vi "AssemblerLauncher.vi"() -> (0 "error out":errorcluster)   [LabVIEW 2017]
uses:
  <vilib>/ActorFramework/Message Enqueuer/Message Priority.ctl
  <vilib>/gpm_packages/@cs/mva-viewable/Source/IViewable/IViewable/View Position Enum.ctl
  <vilib>/gpm_packages/@cs/example/Dynamic Viewables/SequenceSteps/SineModel/SineModel.lvclass
  C:/Program Files/National Instruments/LabVIEW 2017/vi.lib/gpm_packages/@cs/mva-core/Source/IModel/IModel/IModel.lvclass
  <vilib>/gpm_packages/@cs/mva-core/Source/MonitoredMediator/MonitoredMediator/MonitoredMediator.lvclass
  C:/Program Files/National Instruments/LabVIEW 2017/vi.lib/gpm_packages/@cs/mva-core/Source/Mediator/Mediator/Mediator.lvclass
  C:/Program Files/National Instruments/LabVIEW 2017/vi.lib/gpm_packages/@cs/mva-core/Source/IMediator/IMediator/IMediator.lvclass
  <vilib>/gpm_packages/@cs/example/Dynamic Viewables/ViewableChart/ViewableChart.lvclass
  C:/Program Files/National Instruments/LabVIEW 2017/vi.lib/gpm_packages/@cs/mva-viewable/Source/IViewable/IViewable/IViewable.lvclass
  <vilib>/gpm_packages/@cs/example/Dynamic Viewables/ViewableLEDs/ViewableLEDs.lvclass
  <vilib>/gpm_packages/@cs/example/Dynamic Viewables/ViewableButtons/ViewableButtons.lvclass
  <vilib>/gpm_packages/@cs/example/Dynamic Viewables/ViewableStatusBar/ViewableStatusBar.lvclass
  <vilib>/gpm_packages/@cs/example/Dynamic Viewables/SequencingModel/SequencingModel.lvclass
  C:/Program Files/National Instruments/LabVIEW 2017/vi.lib/gpm_packages/@cs/mva-core/Source/IObserver/IObserver/IObserver.lvclass
  <vilib>/gpm_packages/@cs/example/Dynamic Viewables/SequenceSteps/RandomNumberModel/RandomNumberModel.lvclass
  <vilib>/gpm_packages/@cs/example/Dynamic Viewables/SequenceSteps/BlinkyLightModel/BlinkyLightModel.lvclass
  <vilib>/gpm_packages/@cs/example/Dynamic Viewables/ExampleViewModel/ExampleViewModel.lvclass
  C:/Program Files/National Instruments/LabVIEW 2017/vi.lib/gpm_packages/@cs/mva-viewable/Source/IViewModel/IViewModel/IViewModel.lvclass
  C:/Program Files/National Instruments/LabVIEW 2017/vi.lib/ActorFramework/Actor/Actor.lvclass
  <vilib>/gpm_packages/@cs/BusMonitor/ListboxBusMonitor/ListboxBusMonitor/ListboxBusMonitor.lvclass/ListboxBusMonitor.ctl
  <vilib>/gpm_packages/@cs/example/Dynamic Viewables/SequencingModel/SequencingModel.lvclass/SequencingModel.ctl
  <vilib>/gpm_packages/@cs/mva-core/Source/MonitoredMediator/MonitoredMediator/MonitoredMediator.lvclass/MonitoredMediator.ctl
  <vilib>/gpm_packages/@cs/mva-core/Source/Mediator/Mediator/Mediator.lvclass/Mediator.ctl
  <vilib>/gpm_packages/@cs/mva-core/Source/Mediator/TopicLookupTable/TopicLookupTable.lvclass/TopicLookupTable.ctl
  <vilib>/gpm_packages/@cs/mva-core/Source/Mediator/Topic Messages/Add Topic Subscriber Msg/Add Topic Subscriber Msg.lvclass/Add Topic Subscriber Msg.ctl
  <vilib>/ActorFramework/Message Enqueuer/Message Enqueuer.lvclass/Message Enqueuer.ctl
  <vilib>/gpm_packages/@cs/event-logger/Source/Composed Log/LoggerReference/LoggerReference.lvclass/LoggerReference.ctl
  <vilib>/gpm_packages/@cs/mva-core/Source/IObserver/IObserver/IObserver.lvclass/IObserver.ctl
  <vilib>/gpm_packages/@cs/mva-core/Source/IMediator/IMediator/IMediator.lvclass/IMediator.ctl
  <vilib>/gpm_packages/@cs/mva-viewable/Source/IViewModel/IViewModel/IViewModel.lvclass/IViewModel.ctl
  <vilib>/gpm_packages/@cs/mva-viewable/Source/IViewManager/IViewManager Messages/Launch Nested Views Msg/Launch Nested Views Msg.lvclass/Launch Nested Views Msg.ctl
  <vilib>/gpm_packages/@cs/mva-viewable/Source/IViewManager/IViewManager/IViewManager.lvclass/IViewManager.ctl
  <vilib>/gpm_packages/@cs/mva-viewable/Source/IViewable/IViewable Messages/Open Front Panel Msg/Open Front Panel Msg.lvclass/Open Front Panel Msg.ctl
  3903f6a0-0aca-404b-9b59-3d2710bbd38f.vi
  <vilib>/gpm_packages/@cs/mva-core/Source/Mediator/Mediator/Read TopicLookupTable.vi
  <vilib>/gpm_packages/@cs/mva-core/Source/Mediator/TopicLookupTable/Get All Topics.vi
  <vilib>/gpm_packages/@cs/mva-core/Source/Mediator/Topic Messages/Add Topic Subscriber Msg/Send Add Topic Subscriber.vi
  3903f6a0-0aca-404b-9b59-3d2710bbd38f.vi/36d13a4d-583a-4f0f-b811-def87a5d51d4.vi
  <vilib>/gpm_packages/@cs/mva-core/Source/IObserver/IObserver/Configure Observer Logging.vi
  <vilib>/gpm_packages/@cs/mva-viewable/Source/IViewModel/IViewModel/Write Startup Model-View Configuration.vi
  <vilib>/gpm_packages/@cs/mva-core/Source/IMediator/IMediator/Configure Mediator.vi
  <vilib>/ActorFramework/Message Enqueuer/Enqueue.vi
  <vilib>/gpm_packages/@cs/event-logger/Source/Composed Log/LoggerReference/Return Aggregate Queues.vi
  <vilib>/gpm_packages/@cs/event-logger/Source/Composed Log/LoggerReference/Add Aggregate Log.vi
  3903f6a0-0aca-404b-9b59-3d2710bbd38f.vi/36d13a4d-583a-4f0f-b811-def87a5d51d4.vi/bfada182-c8b2-42a6-8ad6-36f5af2b83bc.vi
  <vilib>/gpm_packages/@cs/mva-viewable/Source/IViewManager/IViewManager Messages/Launch Nested Views Msg/Pack Launch Nested Views Msg.vi
  <vilib>/gpm_packages/@cs/mva-viewable/Source/IViewManager/IViewManager/Write Startup Launch Nested Views Msg.vi
  <vilib>/gpm_packages/@cs/event-logger/Source/Composed Log/LoggerReference/Send Add Sink.vi
  <vilib>/gpm_packages/@cs/BusMonitor/ListboxBusMonitor/ListboxBusMonitor/ListboxBusMonitor.lvclass
  C:/Program Files/National Instruments/LabVIEW 2017/vi.lib/gpm_packages/@cs/mva-core/Source/MonitoredMediator/IBusMonitor/IBusMonitor.lvclass
  <vilib>/gpm_packages/@cs/ViewManager/source/BoundViewManager/BoundViewManager.lvclass
  <vilib>/gpm_packages/@cs/mva-core/Source/Mediator/Topic Messages/Add Topic Subscriber Msg/Add Topic Subscriber Msg.lvclass
  C:/Program Files/National Instruments/LabVIEW 2017/vi.lib/ActorFramework/Message/Message.lvclass
  <vilib>/gpm_packages/@cs/event-logger/Source/Text File Sink/Text File Sink.lvclass
  C:/Program Files/National Instruments/LabVIEW 2017/vi.lib/gpm_packages/@cs/event-logger/Source/Composed Log/Log Sink/Log Sink.lvclass
  <vilib>/gpm_packages/@cs/example/Dynamic Viewables/ViewManagerDefaultLayout/ViewManagerDefaultLayout.lvclass
  <vilib>/gpm_packages/@cs/mva-viewable/Source/IViewModel/IViewModel/IViewModel.lvclass
  C:/Program Files/National Instruments/LabVIEW 2017/vi.lib/gpm_packages/@cs/mva-viewable/Source/IViewManager/IViewManager/IViewManager.lvclass
  <vilib>/gpm_packages/@cs/mva-viewable/Source/IViewable/IViewable Messages/Open Front Panel Msg/Open Front Panel Msg.lvclass
  <vilib>/gpm_packages/@cs/mva-core/Source/IMediator/ISubscriptionPolicy/Open Subscription Policy.vi
  <vilib>/ActorFramework/Message Priority Queue/Priority Enqueue.vi
  <vilib>/gpm_packages/@cs/event-logger/Source/Composed Log/Application Logger/Launch Worker Loop.vi
  <vilib>/gpm_packages/@cs/event-logger/Source/Composed Log/LoggerReference/Initialize Logger Instance.vi
  <vilib>/ActorFramework/Message Enqueuer/Message Enqueuer.lvclass
  <vilib>/gpm_packages/@cs/event-logger/Source/Composed Log/LoggerReference/LoggerReference.lvclass
  <vilib>/gpm_packages/@cs/event-logger/Source/Composed Log/IErrorFormat/IErrorFormat.lvclass
  <vilib>/gpm_packages/@cs/event-logger/Source/Composed Log/Log Sink/Log Sink.lvclass
  <vilib>/gpm_packages/@cs/mva-viewable/Source/IViewable/IApplicationStyle/IApplicationStyle.lvclass
  <vilib>/gpm_packages/@cs/mva-viewable/Source/IViewManager/IViewManager Messages/Launch Nested Views Msg/Launch Nested Views Msg.lvclass
  <vilib>/gpm_packages/@cs/mva-core/Source/MonitoredMediator/IBusMonitor/IBusMonitor.lvclass
  <vilib>/ActorFramework/Actor/Actor.lvclass
  <vilib>/gpm_packages/@cs/mva-viewable/Source/IViewable/IViewable/IViewable.lvclass
panel:
  # "Please wait..."
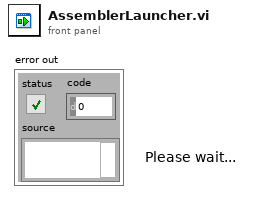
[diagram p1: front panel]
types:
  T1 = typedef "IViewable.lvlib/IViewable.lvclass/View Position Enum.ctl" = enum16{"Centered", "Maximized", "Minimized", "Custom", "Unchanged"}
  T2 = typedef "Actor Framework.lvlib/Message Enqueuer.lvclass/Message Priority.ctl" = enum16{"Low", "Normal", "High"}
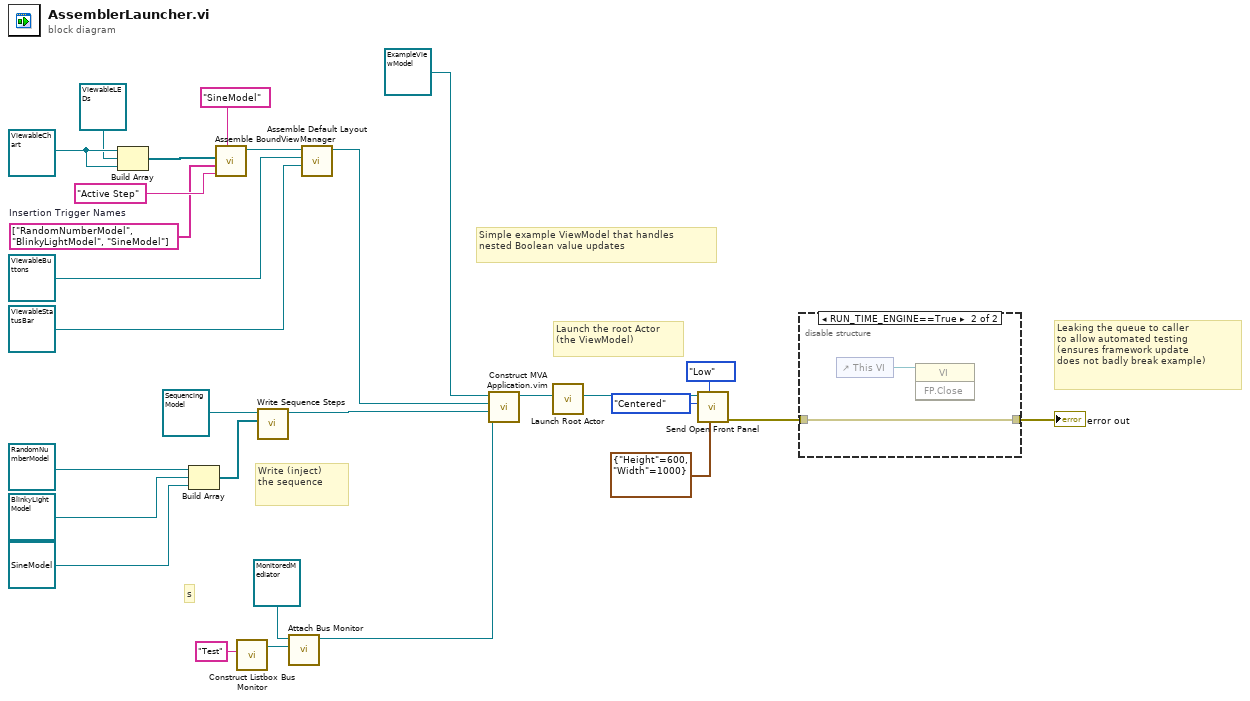
[diagram p0: block diagram]
diagram:
  w7 = string[] ["RandomNumberModel", "BlinkyLightModel", "SineModel"]  # Insertion Trigger Names
  w16 = refnum<class "ViewableChart.lvclass"> refnum ("ViewableChart.lvclass")
  # "s"
  # "Leaking the queue to caller\nto allow automated testing\n(ensures framework update\ndoes not badly break example)"
  # "Write (inject)\nthe sequence"
  # "Launch the root Actor\n(the ViewModel)"
  # "Simple example ViewModel that handles\nnested Boolean value updates"
  n1 = Build Array(w16, refnum<class "ViewableLEDs.lvclass"> refnum ("ViewableLEDs.lvclass"), w16) -> (w9:refnum<class "IViewable.lvclass">[])
  n2 = Build Array(refnum<class "RandomNumberModel.lvclass"> refnum ("RandomNumberModel.lvlib:RandomNumberModel.lvclass"), refnum<class "BlinkyLightModel.lvclass"> refnum ("BlinkyLightModel.lvlib:BlinkyLightModel.lvclass"), refnum<class "SineModel.lvclass"> refnum ("SineModel.lvlib:SineModel.lvclass")) -> (w19:refnum<class "IModel.lvclass">[])
  n3 = call <vilib>:"Assemble BoundViewManager.vi"("Startup View Name (\"\"=None)"="SineModel" ("Startup View Name (\"\"=None)"), "Selector String Name"="Active Step", "Viewable Names"=w7, "Bound Viewables"=w9) -> ("BoundViewManager Out"=w18:refnum<class "BoundViewManager.lvclass">)  [unwired: 7 in]
  n4 = call <vilib>:"Construct Listbox Bus Monitor.vi"("Show Panel Boolean Name"="Test") -> ("ListboxBusMonitor out"=w5:refnum<class "ListboxBusMonitor.lvclass">)  [unwired: 10 in]
  n5 = call <vilib>:"Write Sequence Steps.vi"("Steps"=w19, "SequencingModel in"=refnum<class "SequencingModel.lvclass"> refnum ("SequencingModel.lvlib:SequencingModel.lvclass")) -> ("SequencingModel out"=w20:refnum<class "SequencingModel.lvclass">)  [unwired: 9 in]
  n6 = call <vilib>:"Attach Bus Monitor.vi"("BusMonitor"=w5, "MonitoredMediator in"=refnum<class "MonitoredMediator.lvclass"> refnum ("MonitoredMediator.lvlib:MonitoredMediator.lvclass")) -> ("MonitoredMediator out"=w4:refnum<class "MonitoredMediator.lvclass">)  [unwired: 9 in]
  n7 = call <vilib>:"Assemble Default Layout.vi"("Botom View"=refnum<class "ViewableStatusBar.lvclass"> refnum ("ViewableStatusBar.lvclass"), "Left View"=refnum<class "ViewableButtons.lvclass"> refnum ("ViewableButtons.lvclass"), "Main View"=w18) -> ("ViewManagerDefaultLayout"=w22:refnum<class "ViewManagerDefaultLayout.lvclass">)  [unwired: 8 in]
  n8 = call "Construct MVA Application.vim"("Mediator Type"=w4, "Model Type"=w20, "Startup View Configuration"=w22, "IViewModel In"=refnum<class "ExampleViewModel.lvclass"> refnum ("Dynamic Viewables.lvlib:ExampleViewModel.lvclass")) -> ("IViewModel Out"=w28:refnum<class "ExampleViewModel.lvclass">)  [unwired: 7 in]
  n9 = call <vilib>:"Launch Root Actor.vi"("Actor"=w28) -> ("Actor's Enqueuer"=w27:refnum<class "Message Enqueuer.lvclass">)  [unwired: 9 in, 1 out]
  n10 = call <vilib>:"Send Open Front Panel.vi"("Custom Window Size"=cluster{"Height":i16, "Width":i16} {"Height"=600, "Width"=1000}, "Message Priority (Normal)"=Message_Priority."Low", "Position"=View_Position_Enum."Centered", "Message Enqueuer"=w27) -> ("error out"=w24:errorcluster)  [unwired: 6 in, 1 out]
  n11 = disable-structure shown="RUN_TIME_ENGINE==True" {
    disable-tunnel: w24 -> [w29 w31]
    disable-tunnel: [w29 w31] -> w23
    frame condition #0 (active) {
    }
    frame condition #1 {
      n12 = control-ref of="This VI"() -> (w30:refnum<vi>)
      n13 = invoke class="VI" method="FP.Close"(reference=w30) -> ()  [unwired: 2 in, 3 out]
    }
  }
  "error out" <- w23
